vi "Test Helper Loop Errors sent to Error Handler.vi"(8 "error in (no error)":errorcluster, 11 "Helper Loop Test In":refnum<class "Helper Loop Test.lvclass">) -> (0 "error out":errorcluster, 3 "Helper Loop Test Out":refnum<class "Helper Loop Test.lvclass">)   [LabVIEW 2020, in "Helper Loop Test.lvclass"]
uses:
  Helper Loop Test.lvclass
  C:/Program Files (x86)/National Instruments/LabVIEW 2020/vi.lib/Asteme/LUnit/Test Case.lvclass
  Mock Process/Mock Process.lvclass
  C:/Users/anton/Documents/GitHub/Triarc-Framework/source/Framework/Process/Process.lvclass
  Mock Error Handler/Mock Error Handler.lvclass
  C:/Users/anton/Documents/GitHub/Triarc-Framework/source/Framework/Error Handler Interface/Error Handler Interface.lvclass
  Framework/Process/Process.lvclass/Process.ctl
  <vilib>/Asteme/LUnit/Test Case.lvclass/Test Case.ctl
  <vilib>/Asteme/LUnit/LUnit Assertion Result.lvclass/LUnit Assertion Result.ctl
  Framework/Process/Protected/Messaging/Enqueue Message.vi
  Framework/Process/Public/Lifecycle/Get Lifecycle State.vi
  <vilib>/Utility/error.llb/Clear Errors.vi
  <vilib>/Asteme/LUnit/Palette/Pass.vi
  <vilib>/Asteme/LUnit/Palette/Fail.vi
  <vilib>/Asteme/LUnit/Variant to string.vi
  <vilib>/Asteme/LUnit/Set Assertion Type.vi
  Framework/Process/Private/SubVIs/Wait for finish.vi
  Framework/Process/Private/SubVIs/Set Lifecycle State.vi
  <vilib>/Asteme/LUnit/Add test result.vi
  <vilib>/Asteme/LUnit/LUnit Write Passed.vi
  <vilib>/Asteme/LUnit/LUnit Get Test Case.vi
  <vilib>/Asteme/LUnit/Assertion Result/LUnit Get Test Name.vi
  <vilib>/Asteme/LUnit/LUnit Write Message.vi
  <vilib>/Asteme/LUnit/LUnit Write Description.vi
  <vilib>/Asteme/LUnit/LUnit Write Assertion Type.vi
  <vilib>/Asteme/LUnit/Read Test Case Name.vi
  <vilib>/Utility/error.llb/Error Cluster From Error Code.vi
  <vilib>/Utility/Data Type/Get Type Information.vi
  <vilib>/Utility/LVClass/Get LV Class Name.vi
  Framework/Process/Process.lvclass
  <vilib>/Asteme/LUnit/LUnit Assertion Result.lvclass
  <vilib>/Asteme/LUnit/Test Case.lvclass
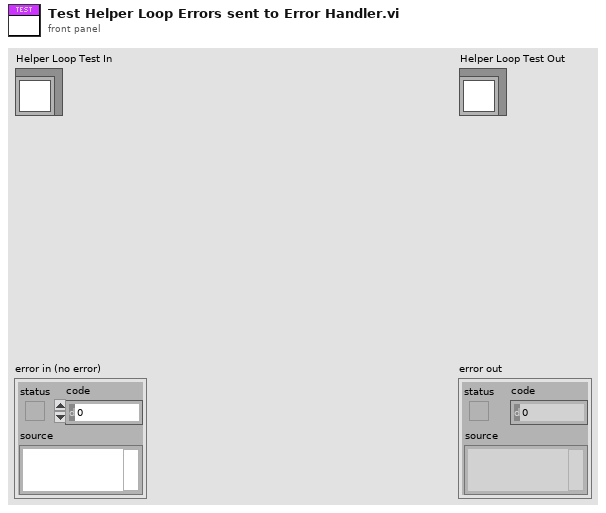
[diagram p1: front panel]
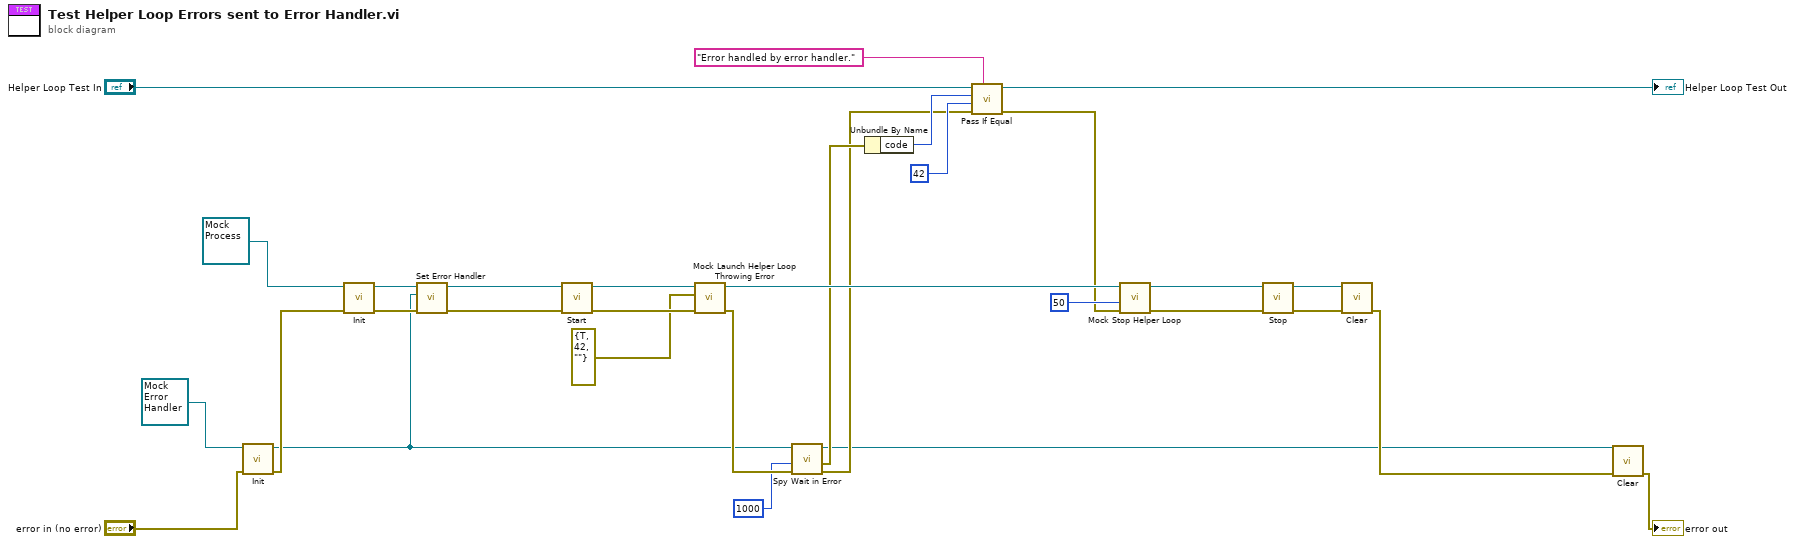
[diagram p0: block diagram]
diagram:
  n1 = call-dynamic "Init.vi"("error in (no error)"="error in (no error)", "Mock Error Handler In"=refnum<class "Mock Error Handler.lvclass"> refnum) -> ("error out"=w4:errorcluster, "Mock Error Handler Out"=w3:refnum<class "Mock Error Handler.lvclass">)  [unwired: 8 in]
  n2 = call-dynamic "Init.vi"("error in (no error)"=w4, "Mock Process In"=refnum<class "Mock Process.lvclass"> refnum) -> ("error out"=w19:errorcluster, "Mock Process Out"=w31:refnum<class "Mock Process.lvclass">)  [unwired: 8 in]
  n3 = call "Set Error Handler.vi"("error in (no error)"=w19, "Error Handler"=w3, "Process In"=w31) -> ("error out"=w18:errorcluster, "Process Out"=w20:refnum<class "Mock Process.lvclass">)  [unwired: 7 in]
  n4 = call "Start.vi"("error in (no error)"=w18, "Process In"=w20) -> ("error out"=w29:errorcluster, "Process Out"=w30:refnum<class "Mock Process.lvclass">)  [unwired: 8 in]
  n5 = call "Mock Launch Helper Loop Throwing Error.vi"("error in (no error)"=w29, "Error message"=errorcluster {"status"=TRUE, "code"=42, "source"=""}, "Mock Process in"=w30) -> ("error out"=w15:errorcluster, "Mock Process out"=w28:refnum<class "Mock Process.lvclass">)  [unwired: 7 in]
  n6 = call "Spy Wait in Error.vi"("error in (no error)"=w15, "timeout in ms (-1)"=1000, "Mock Error Handler In"=w3) -> ("error out"=w5:errorcluster, "Errors"=w9:errorcluster, "Mock Error Handler Out"=w2:refnum<class "Mock Error Handler.lvclass">)  [unwired: 4 in, 2 out]
  n7 = Unbundle By Name(w9) -> ("code"=w8:i32)
  n8 = call <vilib>:"Pass If Equal.vi"("Description"="Error handled by error handler.", "error in (no error)"=w5, "Actual"=42 ("code"), "Expected"=w8, "Test Case In"="Helper Loop Test In") -> ("error out"=w11:errorcluster, "Test Case Out"=→"Helper Loop Test Out":refnum<class "Helper Loop Test.lvclass">)  [unwired: 5 in]
  n9 = call "Mock Stop Helper Loop.vi"("error in (no error)"=w11, "timeout in ms (-1)"=50, "Mock Process in"=w28) -> ("error out"=w26:errorcluster, "Mock Process out"=w27:refnum<class "Mock Process.lvclass">)  [unwired: 6 in, 1 out]
  n10 = call "Stop.vi"("error in (no error)"=w26, "Process In"=w27) -> ("error out"=w25:errorcluster, "Process Out"=w1:refnum<class "Mock Process.lvclass">)  [unwired: 7 in, 1 out]
  n11 = call-dynamic "Clear.vi"("error in (no error)"=w25, "Mock Process In"=w1) -> ("error out"=w24:errorcluster)  [unwired: 9 in]
  n12 = call-dynamic "Clear.vi"("error in (no error)"=w24, "Mock Process In"=w2) -> ("error out"=→"error out":errorcluster)  [unwired: 9 in]
